vi "niDAQmx Create Virtual Channel (Digital Output).vi"(0 "task in":refnum<class "Session Factory.lvclass">, 5 "lines":tag, 7 "name to assign":string, 9 "line grouping":i32(ring)=1 items=["one channel for each line", "one channel for all lines"], 11 "error in":errorcluster) -> (4 "task out":refnum<class "Session Factory.lvclass">, 15 "error out":errorcluster)   [LabVIEW 2021, in "Session Management niDAQmx.lvlib" / "Session Factory.lvclass"]
doc: "Creates channel(s) to generate digital signals. You can group digital lines into one digital channel or separate them into multiple digital channels. If you specify one or more entire ports in lines input by using port physical channel names, you cannot separate the ports into multiple channels. To separate ports into multiple channels, use this VI multiple times with a different port each time."
uses:
  Session Factory.lvclass
  NI_DAQmx_client/RPC Messages/nidaqmx_grpc_CreateDOChanRequest.ctl
  NI_DAQmx_client/RPC Messages/nidevice_grpc_Session.ctl
  NI_DAQmx_client/RPC Messages/nidevice_grpc_Session_session/nidevice_grpc_Session_session.lvclass
  NI_DAQmx_client/RPC Messages/nidaqmx_grpc_CreateDOChanRequest_line_grouping_enum/nidaqmx_grpc_CreateDOChanRequest_line_grouping_enum.lvclass
  Session Factory.lvclass/Session Factory.ctl
  NI_DAQmx_client/RPC Messages/nidaqmx_grpc_LineGrouping.ctl
  NI_DAQmx_client/RPC Messages/nidaqmx_grpc_CreateDOChanRequest_line_grouping_enum/nidaqmx_grpc_CreateDOChanRequest_line_grouping_enum.lvclass/nidaqmx_grpc_CreateDOChanRequest_line_grouping_enum.ctl
  NI_DAQmx_client/NI_DAQmx_client.lvlib
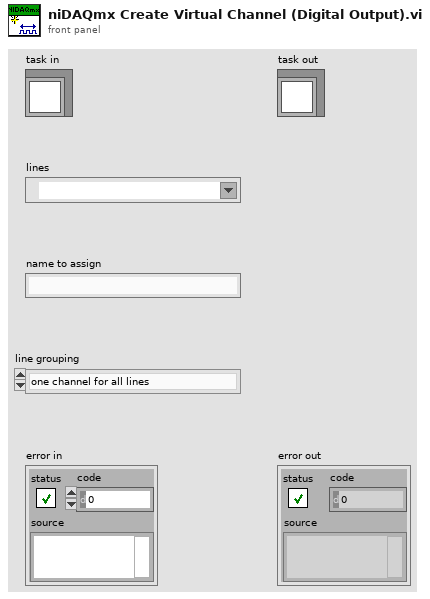
[diagram p1: front panel]
types:
  T1 = typedef "NI_DAQmx_client.lvlib/nidaqmx_grpc_CreateDOChanRequest.ctl" = cluster{"task":T2, "lines":string, "name_to_assign_to_lines":string, "nidaqmx_grpc_CreateDOChanRequest_line_grouping_enum":refnum<class "nidaqmx_grpc_CreateDOChanRequest_line_grouping_enum.lvclass">}
  T2 = typedef "NI_DAQmx_client.lvlib/nidevice_grpc_Session.ctl" = cluster{"nidevice_grpc_Session_session":refnum<class "nidevice_grpc_Session_session.lvclass">}
  T3 = typedef "NI_DAQmx_client.lvlib/nidaqmx_grpc_LineGrouping.ctl" = enum32{"LINE_GROUPING_CHAN_PER_LINE", "LINE_GROUPING_CHAN_FOR_ALL_LINES"}
  T4 = typedef "grpc-lvsupport-release.lvlib/grpcId.ctl" = u64
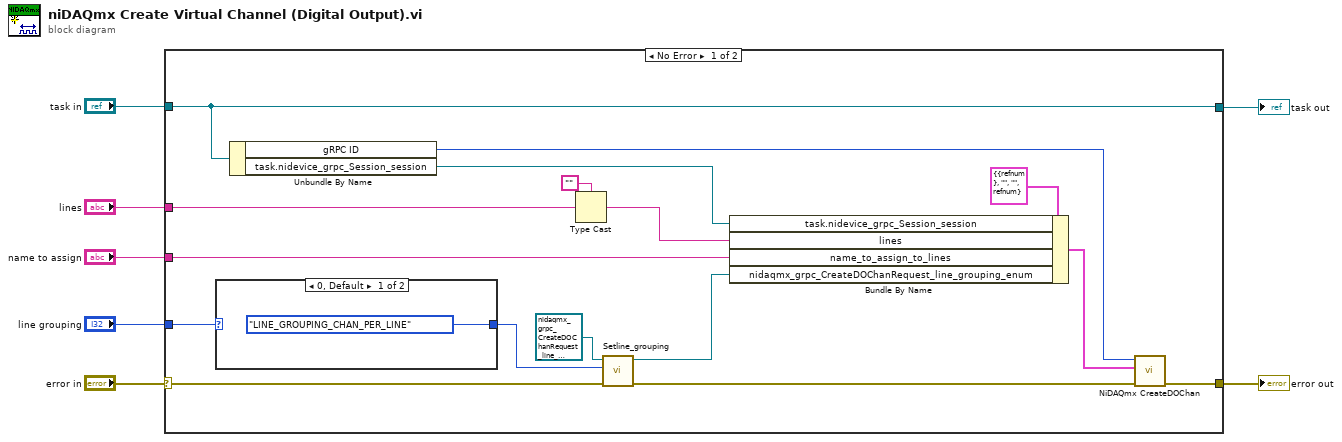
[diagram p0: block diagram]
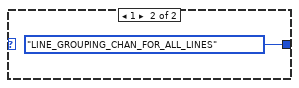
[diagram p2: hidden frame]
diagram:
  n1 = case shown="No Error" "error in" {
    selector: "error in" -> [w13 w27]
    tunnel: [w23 w27] -> w6
    tunnel: "task in" -> [w22 w26]
    tunnel: [w22 w26] -> w4
    tunnel: "lines" -> [w17 _]
    tunnel: "name to assign" -> [w14 _]
    tunnel: "line grouping" -> [w10 _]
    frame No Error {
      n2 = case shown="0, Default" w10 {
        tunnel: [nidaqmx_grpc_LineGrouping."LINE_GROUPING_CHAN_PER_LINE" ("Set_Val") nidaqmx_grpc_LineGrouping."LINE_GROUPING_CHAN_FOR_ALL_LINES" ("Set_Val")] -> w9
        frame 0, Default {
        }
        frame 1 {
        }
      }
      n3 = Unbundle By Name(w22) -> ("gRPC ID"=w21:T4, "task.nidevice_grpc_Session_session"=w18:refnum<class "nidevice_grpc_Session_session.lvclass">)
      n4 = Type Cast(type="", x=w17) -> (*(type *) &x=w15:string)
      n5 = call "Setline_grouping.vi"("error in (no error)"=w13, "Set_Val"=w9, "OneOfTemplate in"=refnum<class "nidaqmx_grpc_CreateDOChanRequest_line_grouping_enum.lvclass"> refnum) -> ("error out"=w12:errorcluster, "OneOfTemplate out"=w11:refnum<class "nidaqmx_grpc_CreateDOChanRequest_line_grouping_enum.lvclass">)  [unwired: 7 in]
      n6 = Bundle By Name(cluster=T1 {"task"={"nidevice_grpc_Session_session"=refnum}, "lines"="", "name_to_assign_to_lines"="", "nidaqmx_grpc_CreateDOChanRequest_line_grouping_enum"=refnum} ("Request Data"), "task.nidevice_grpc_Session_session"=w18, "lines"=w15, "name_to_assign_to_lines"=w14, "nidaqmx_grpc_CreateDOChanRequest_line_grouping_enum"=w11) -> (w19:T1)
      n7 = call "NiDAQmx CreateDOChan.vi"("error in"=w12, "Request Data"=w19, "gRPC ID"=w21) -> ("error out"=w23:errorcluster)  [unwired: 6 in, 2 out]
    }
    frame Error {
    }
  }
  "error out" <- w6
  "task out" <- w4
